vi "Initialize Transfer.vi"(7 "id":i32, 8 "error in (no error)":errorcluster, 9 "convert (F)":bool, 10 "Buffers":refnum<class "Buffers.lvclass">, 11 "Transfer Configuration":T1 {"channels"."string offset" format="%d bytes"}) -> (0 "error out":errorcluster, 3 "Transfer out":refnum<class "Transfer.lvclass">)   [LabVIEW 2017, in "DSF Core.lvlib" / "Transfer.lvclass"]
uses:
  Transfer.lvclass
  Typedefs/DSF Engine Transfer Configuration.ctl
  Typedefs/DSF Byte Order.ctl
  Typedefs/DSF Settings Info.ctl
  Typedefs/DSF Engine Channel Configuration.ctl
  Typedefs/DSF Data Type.ctl
  Buffers/Buffers.lvclass
  Transfer.lvclass/Transfer.ctl
  DSF Core.lvlib
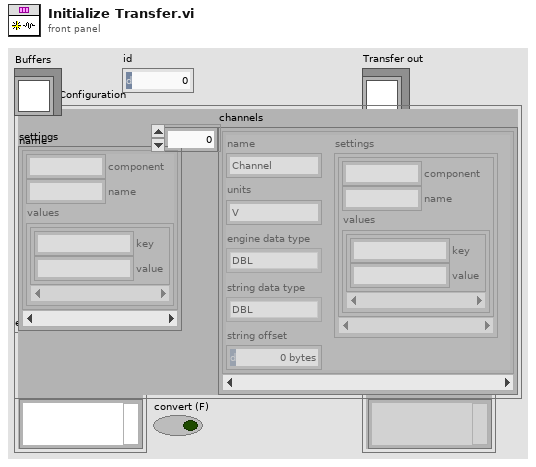
[diagram p1: front panel]
types:
  T1 = typedef "DSF Core.lvlib/DSF Engine Transfer Configuration.ctl" = cluster{"name":string, "byte order":T2, "settings":T3, "channels":T4[]}
  T2 = typedef "DSF Core.lvlib/DSF Byte Order.ctl" = enum8{"big-endian", "little-endian"}
  T3 = typedef "DSF Core.lvlib/DSF Settings Info.ctl" = cluster{"component":string, "name":string, "values":cluster{"key":string, "value":string}[]}[]
  T4 = typedef "DSF Core.lvlib/DSF Engine Channel Configuration.ctl" = cluster{"string offset":u64, "name":string, "units":string, "engine data type":T5, "string data type":T5, "settings":T3}
  T5 = typedef "DSF Core.lvlib/DSF Data Type.ctl" = enum8{"Bool", "SGL", "DBL", "I8", "I16", "I32", "I64", "U8", "U16", "U32", "U64"}
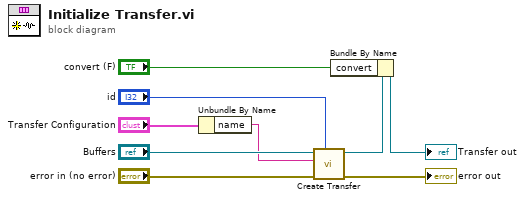
[diagram p0: block diagram]
diagram:
  n1 = Unbundle By Name("Transfer Configuration") -> ("name"=w4:string)
  n2 = call "Create Transfer.vi"("id"="id", "error in (no error)"="error in (no error)", "name"=w4, "Buffers"="Buffers") -> ("error out"=→"error out":errorcluster, "Transfer out"=w3:refnum<class "Transfer.lvclass">)  [unwired: 6 in]
  n3 = Bundle By Name(cluster=w3, "convert"="convert (F)") -> (→"Transfer out":refnum<class "Transfer.lvclass">)
